vi "insert_me.vi"(8 "error in (no error)":errorcluster, 11 "DataCollectionDL110128Streaming in":refnum<class "DataCollectionDL110128Streaming.lvclass">) -> (0 "error out":errorcluster, 3 "DataCollectionDL110128Streaming out":refnum<class "DataCollectionDL110128Streaming.lvclass">)   [LabVIEW 2010, in "DataCollectionDL110128Streaming.lvclass"]
uses:
  DataCollectionDL110128Streaming.lvclass
  common/classes/GenericComponent/GenericComponent/class_data.vi
  common/classes/GenericComponent/GenericComponent/GenericComponent.lvclass
panel:
  out "appended path":path
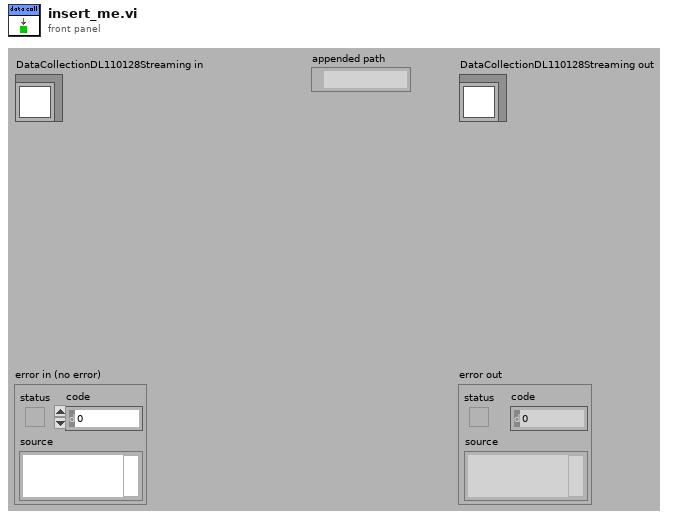
[diagram p1: front panel]
types:
  T1 = enum16{"open", "replace", "create", "open or create", "replace or create", "replace or create with confirmation"}
  T2 = typedef "pixel_raw_data_array.ctl" = dbl[][]
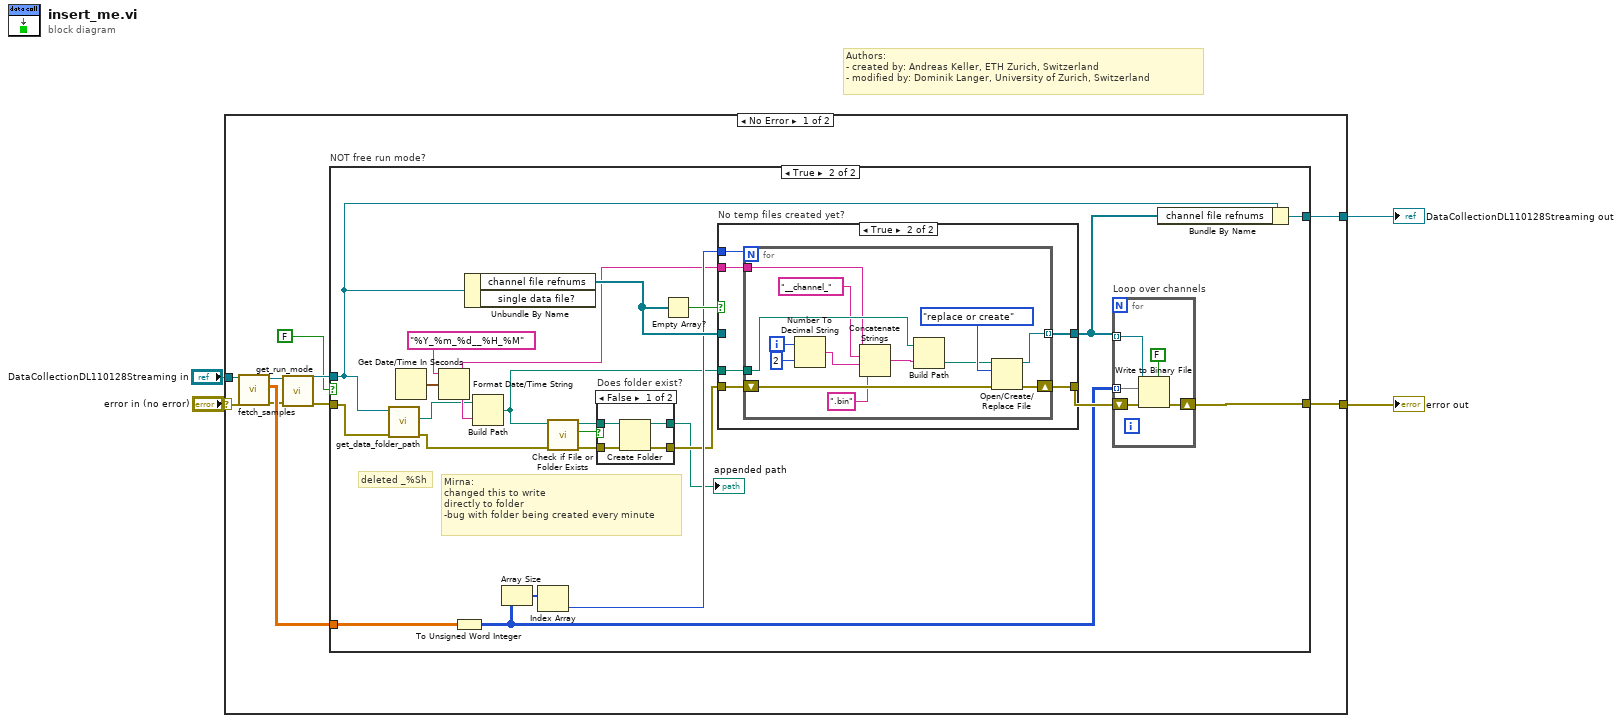
[diagram p0: block diagram]
diagram:
  # "Authors: \n- created by: Andreas Keller, ETH Zurich, Switzerland\n- modified by: Dominik Langer, University of Zurich, Switzerland"
  n1 = case shown="No Error" "error in (no error)" {
    selector: "error in (no error)" -> [w13 w73]
    tunnel: [w12 w73] -> w3
    tunnel: [w11 w72] -> w1
    tunnel: "DataCollectionDL110128Streaming in" -> [w14 w72]
    frame No Error {
      n2 = call-dynamic "fetch_samples.vi"("error in (no error)"=w13, "GenericToplevelComponent in"=w14) -> ("error out"=w9:errorcluster, "channels raw data block"=w10:T2, "GenericToplevelComponent out"=w7:refnum<class "DataCollectionDL110128Streaming.lvclass">)  [unwired: 6 in, 1 out]
      n3 = call "get_run_mode.vi"("error in (no error)"=w9, "GenericPlugin in"=w7) -> ("error out"=w8:errorcluster, "GenericPlugin out"=w6:refnum<class "DataCollectionDL110128Streaming.lvclass">)  [unwired: 5 in, 3 out]
      n4 = case "NOT free run mode?" shown="True" FALSE {
        tunnel: [w16 w26] -> w12
        tunnel: [w15 w37] -> w11
        tunnel: w10 -> [_ w35]
        tunnel: w8 -> [w16 w29]
        tunnel: w6 -> [w15 w28]
        frame False {
        }
        frame True {
          # "Mirna:\nchanged this to write\ndirectly to folder\n-bug with folder being created every minute"
          # "deleted _%Sh"
          n5 = call-dynamic "get_data_folder_path.vi"("error in (no error)"=w29, "GenericComponent in"=w28) -> ("error out"=w21:errorcluster, "data folder path"=w17:path)  [unwired: 8 out]
          n6 = Get Date/Time In Seconds() -> (seconds since 1Jan1904=w30:timestamp)
          n7 = Format Date/Time String(time format string (%c)="%Y_%m_%d__%H_%M", seconds (now)=w30) -> (date/time string=w25:string)  [unwired: 1 out]
          n8 = To Unsigned Word Integer(number=w35) -> (unsigned 16bit integer=w34:u16[][])
          n9 = Unbundle By Name(w28) -> ("channel file refnums"=w39:refnum<file>[])  [unwired: 1 out]
          n10 = Build Path(base path=w17, name or relative path=w25) -> (appended path=w22:path)
          n11 = Array Size(array=w34) -> (size(s)=w33:i32[])
          n12 = Index Array(array=w33) -> (element=w32:i32)  [unwired: 1 in]
          n13 = call <vilib>:"Check if File or Folder Exists.vi"("error in (no error)"=w21, "path"=w22) -> ("error out"=w24:errorcluster, "file or folder exists?"=w23:bool, "dup path"=w20:path)  [unwired: 7 in]
          n14 = case "Does folder exist?" shown="False" w23 {
            tunnel: w20 -> [w43 w44]
            tunnel: w24 -> [w42 w45]
            tunnel: [w41 w45] -> w19
            tunnel: [w40 w44] -> w18
            frame False {
              n15 = Create Folder(path (use dialog)=w43, error in=w42) -> (created path=w40:path, error out=w41:errorcluster)  [unwired: 1 in, 1 out]
            }
            frame True {
            }
          }
          "appended path" <- w18
          n16 = Empty Array?(array=w39) -> (empty?=w36:bool)
          n17 = case "No temp files created yet?" shown="True" w36 {
            tunnel: w19 -> [w52 w58]
            tunnel: [w52 w57] -> w38
            tunnel: w39 -> [w51 _]
            tunnel: [w51 w56] -> w27
            tunnel: w32 -> [_ w55]
            tunnel: w22 -> [_ w54]
            tunnel: w25 -> [_ w53]
            frame False {
            }
            frame True {
              n18 = for {
                N: w55 -> [_]
                shift-right: [w71] -> w57
                shift-left: w58 -> [w65]
                tunnel: [w70] -> w56 mode=indexing
                tunnel: w54 -> [w64]
                tunnel: w53 -> [w60]
                i -> [w67]
                n19 = Number To Decimal String(number=w67, width (-)=i16 2) -> (decimal integer string=w61:string)
                n20 = Concatenate Strings(w60, "__channel_" ("string"), w61, ".bin" ("string")) -> (w59:string)
                n21 = Build Path(base path=w64, name or relative path=w59) -> (appended path=w68:path)
                n22 = Open/Create/Replace File(file path (use dialog)=w68, error in=w65, operation (0:open)=T1."replace or create") -> (refnum out=w70:refnum<file>, error out=w71:errorcluster)  [unwired: 3 in, 1 out]
              }
            }
          }
          n23 = for "Loop over channels" {
            tunnel: w27 -> [w48] mode=indexing
            tunnel: w34 -> [w46] mode=indexing
            shift-right: [w49] -> w26
            shift-left: w38 -> [w50]
            n24 = Write to Binary File(file (use dialog)=w48, data=w46, error in=w50, 5:FALSE ("prepend array or string size? (T)")) -> (error out=w49:errorcluster)  [unwired: 2 in, 2 out]
          }
          n25 = Bundle By Name(cluster=w28, "channel file refnums"=w27) -> (w37:refnum<class "DataCollectionDL110128Streaming.lvclass">)
        }
      }
    }
    frame Error {
    }
  }
  "error out" <- w3
  "DataCollectionDL110128Streaming out" <- w1
